vi "FeedbackDecode_GetPupilInfo.vi"(3 "FullDataPath":path=path "D:/FeedbackDecode/00000000-000000") -> ()   [LabVIEW 2020]
uses:
  <vilib>/addons/zeromq/socket_type.ctl
  <vilib>/addons/zeromq/socket_options.ctl
  <vilib>/DAQmx/write.llb/DAQmx Write (Analog DBL 1Chan 1Samp).vi
  FeedbackDecode_Globals.vi
  <vilib>/DAQmx/miscellaneous.llb/DAQmx Fill In Error Info.vi
  <vilib>/addons/zeromq/zeromq.lvlib
  <vilib>/addons/zeromq/zmq_context.lvclass
  <vilib>/addons/zeromq/zmq_socket.lvclass
panel:
  out "PupilDia":dbl
  out "PupilClust":T1
  out "error out":errorcluster
  out "RecStatus":string
  out "FileTime":string
  out "DataFolderName":string="00000000-000000"
  out "SubPort":string
  out "Acquire":dbl(graph)
  out "message":string[](array[string])
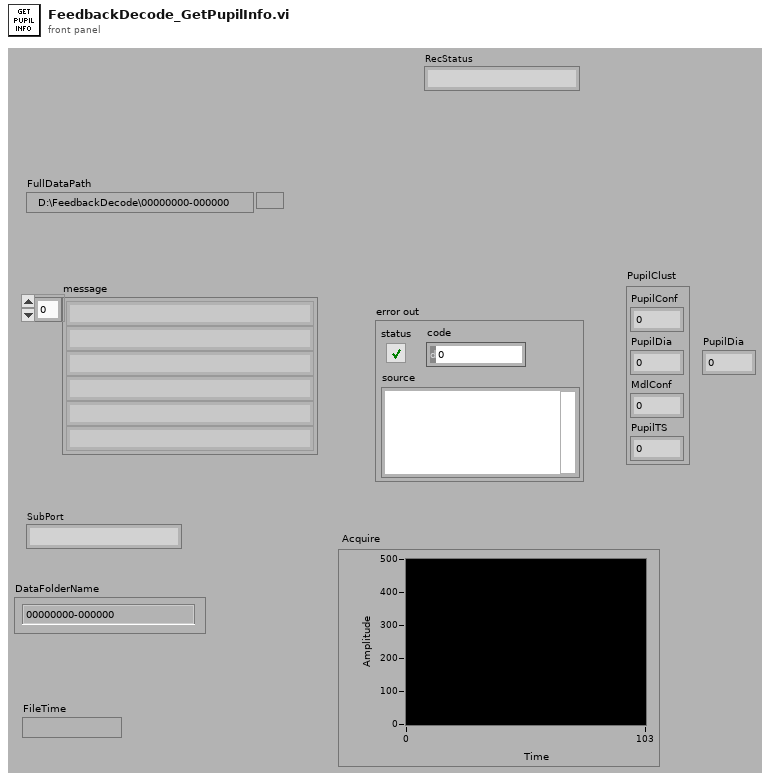
[diagram p1: front panel]
types:
  T1 = cluster{"PupilConf":dbl, "PupilDia":dbl, "MdlConf":dbl, "PupilTS":dbl}
  T2 = typedef "zeromq.lvlib/socket_options.ctl" = enum8{"NONE", "ZMQ_HWM", "<2>", "ZMQ_SWAP", "ZMQ_AFFINITY", "ZMQ_IDENTITY", "ZMQ_SUBSCRIBE", "ZMQ_UNSUBSCRIBE", "ZMQ_RATE", "ZMQ_RECOVERY_IVL", "ZMQ_MCAST_LOOP", "ZMQ_SNDBUF", "ZMQ_RCVBUF", "ZMQ_RCVMORE", "ZMQ_FD", "ZMQ_EVENTS", "ZMQ_TYPE", "ZMQ_LINGER", "ZMQ_RECONNECT_IVL", "ZMQ_BACKLOG", "ZMQ_RECOVERY_IVL_MSEC", "ZMQ_RECONNECT_IVL_MAX", "ZMQ_MAXMSGSIZE", "ZMQ_SNDHWM", "ZMQ_RCVHWM", "ZMQ_MULTICAST_HOPS", "<26>", "ZMQ_RCVTIMEO", "ZMQ_SNDTIMEO", "<29>", "<30>", "ZMQ_IPV4ONLY", "ZMQ_LAST_ENDPOINT", "ZMQ_ROUTER_MANDATORY", "ZMQ_TCP_KEEPALIVE", "ZMQ_TCP_KEEPALIVE_CNT", "ZMQ_TCP_KEEPALIVE_IDLE", "ZMQ_TCP_KEEPALIVE_INTVL", "ZMQ_TCP_ACCEPT_FILTER", "ZMQ_DELAY_ATTACH_ON_CONNECT", "ZMQ_XPUB_VERBOSE"}
  T3 = typedef "zeromq.lvlib/socket_type.ctl" = enum8{"ZMQ_PAIR", "ZMQ_PUB", "ZMQ_SUB", "ZMQ_REQ", "ZMQ_REP", "ZMQ_DEALER", "ZMQ_ROUTER", "ZMQ_PULL", "ZMQ_PUSH", "ZMQ_XPUB", "ZMQ_XSUB"}
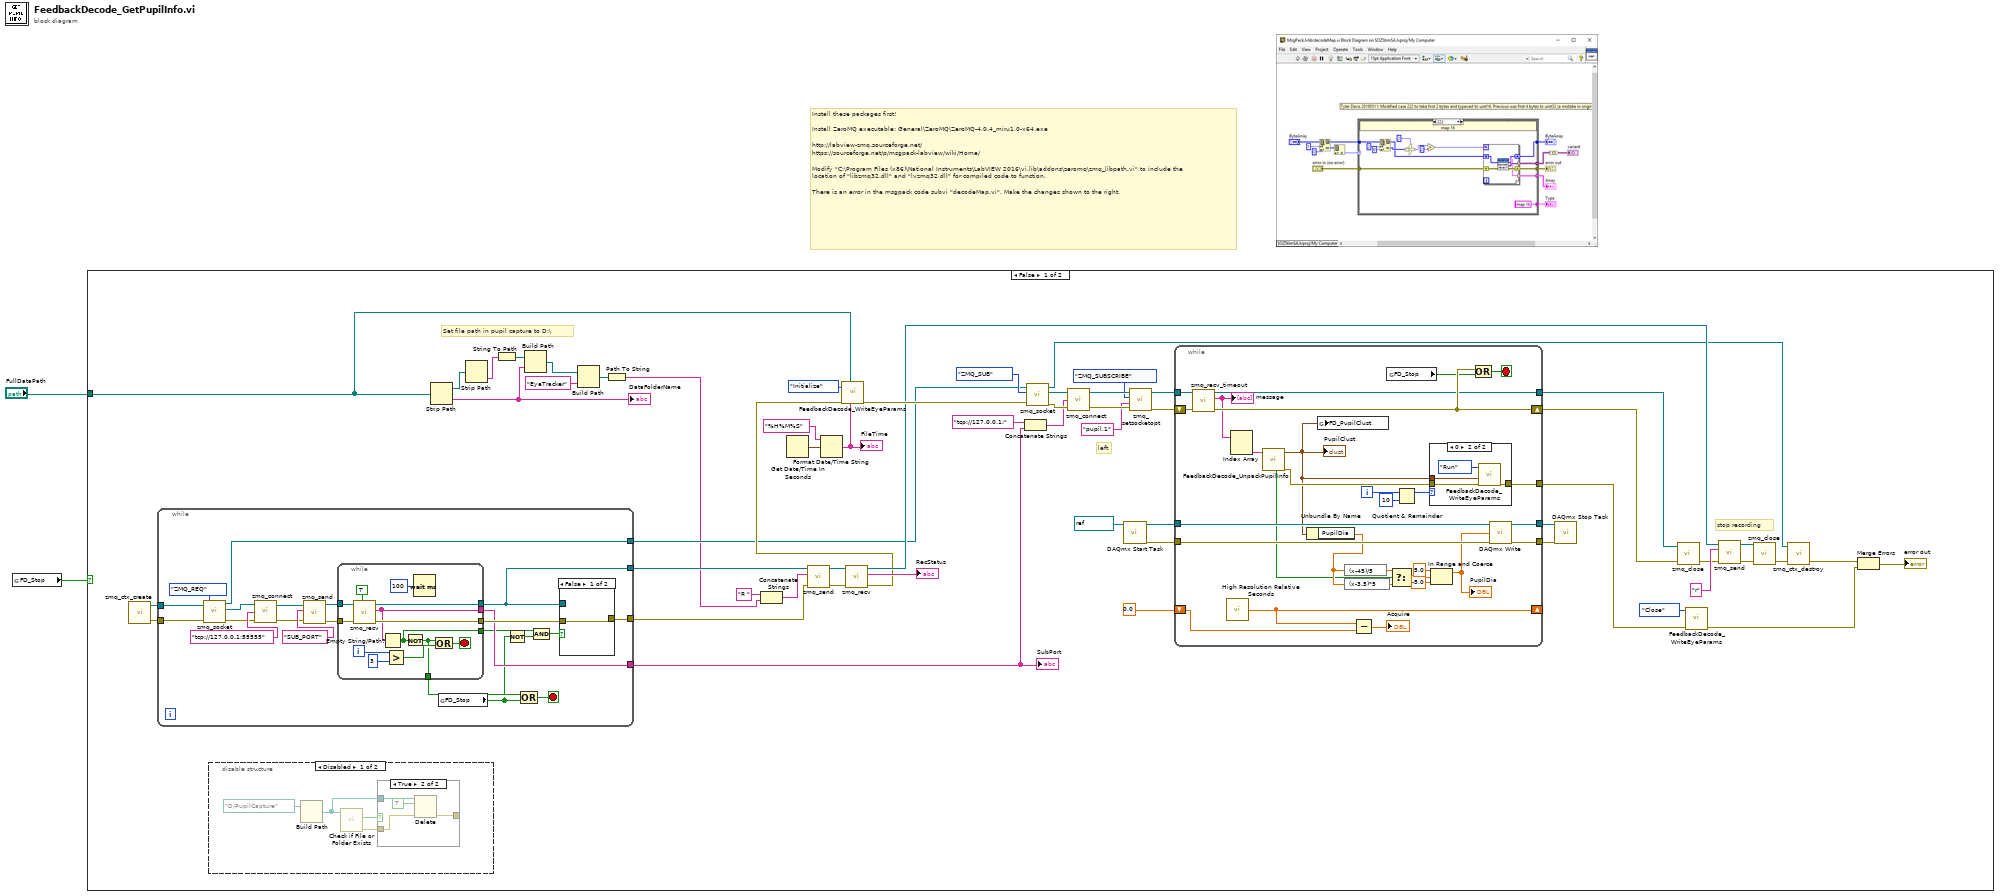
[diagram p0: block diagram]
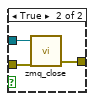
[diagram p2: hidden frame]
diagram:
  # "Install these packages first!\n\nInstall ZeroMQ executable: General\\ZeroMQ\\ZeroMQ-4.0.4_miru1.0-x64.exe\n\nhttp://labview-zmq.sourceforge.net/\nhttps://sourceforge.net/p/msgpack-labview/wiki/Home/\n\nModify \"C:\\Program Files (x86)\\National Instruments\\LabVIEW 2016\\vi.lib\\addons\\zeromq\\zmq_libpath.vi\" to include the location of \"libzmq32.dll\" and \"lvzmq32.dll\" for compiled code to function.\n\nThere is an error in the msgpack code subvi \"decodeMap.vi\". Make the changes shown to the right."
  n1 = global read "FeedbackDecode_Globals.vi" "FD_Stop"() -> (w1:bool)
  n2 = case shown="False" w1 {
    tunnel: "FullDataPath" -> [w5 _]
    frame False {
      # "Set file path in pupil capture to D:\\"
      # "left"
      # "stop recording"
      n3 = call <vilib>:"zmq_ctx_create.vi"() -> ("error out"=w21:errorcluster, "context out"=w22:refnum<class "zmq_context.lvclass">)  [unwired: 4 in]
      n4 = while {
        tunnel: [w72] -> w24
        tunnel: [w71] -> w23
        tunnel: [w67] -> w25
        tunnel: [w66] -> w20
        tunnel: w21 -> [w65]
        tunnel: w22 -> [w64]
        stop <- w78 stop-if-true
        n5 = call <vilib>:"zmq_socket.vi"("error in"=w65, "socket type"=socket_type."ZMQ_REQ", "context in"=w64) -> ("error out"=w69:errorcluster, "socket out"=w68:refnum<class "zmq_socket.lvclass">, "context out"=w66:refnum<class "zmq_context.lvclass">)  [unwired: 2 in]
        n6 = call <vilib>:"zmq_connect.vi"("error in"=w69, "endpoint"="tcp://127.0.0.1:55555", "socket in"=w68) -> ("error out"=w74:errorcluster, "socket out"=w75:refnum<class "zmq_socket.lvclass">)  [unwired: 1 in]
        n7 = call <vilib>:"zmq_send.vi"("error in"=w74, "data"="SUB_PORT", "socket in"=w75) -> ("error out"=w80:errorcluster, "socket out"=w79:refnum<class "zmq_socket.lvclass">)  [unwired: 4 in]
        n8 = while {
          tunnel: [w89] -> w71
          tunnel: [w87] -> w77
          tunnel: w79 -> [w97]
          tunnel: [w96] -> w67
          tunnel: w80 -> [w98]
          tunnel: [w95] -> w73
          tunnel: [w86] -> w63
          i -> [w90]
          stop <- w91 stop-if-true
          n9 = call <vilib>:"zmq_recv.vi"("no block? (F)"=TRUE, "error in"=w98, "socket in"=w97) -> ("error out"=w95:errorcluster, "data"=w89:string, "socket out"=w96:refnum<class "zmq_socket.lvclass">)  [unwired: 2 in, 2 out]
          n10 = Empty String/Path?(string/path=w89) -> (empty?=w86:bool)
          n11 = Greater?(x=w90, y=3) -> (0:w88:bool)
          n12 = Not(x=w86) -> (.not. x?=w87:bool)
          n13 = Wait (ms)(milliseconds to wait=u32 100) -> ()  [unwired: 1 out]
          n14 = Compound Arithmetic op=OR(w87, w88) -> (w91:bool)
        }
        n15 = global read "FeedbackDecode_Globals.vi" "FD_Stop"() -> (w60:bool)
        n16 = Not(x=w60) -> (.not. x?=w62:bool)
        n17 = Compound Arithmetic op=OR(w77, w60) -> (w78:bool)
        n18 = Compound Arithmetic op=AND(w63, w62) -> (w61:bool)
        n19 = case shown="False" w61 {
          tunnel: w67 -> [_ w85]
          tunnel: w73 -> [w82 w84]
          tunnel: [w82 w83] -> w72
          frame False {
          }
          frame True {
            n20 = call <vilib>:"zmq_close.vi"("error in"=w84, "socket"=w85) -> ("error out"=w83:errorcluster)  [unwired: 3 in]
          }
        }
      }
      "SubPort" <- w23
      n21 = disable-structure shown="Disabled" {
        frame Disabled {
          n22 = Build Path(base path=path "D:/PupilCapture") -> (appended path=w100:path)  [unwired: 1 in]
          n23 = call <vilib>:"Check if File or Folder Exists.vi"("path"=w100) -> ("error out"=w99:errorcluster, "file or folder exists?"=w101:bool)  [unwired: 8 in, 1 out]
          n24 = case shown="True" w101 {
            tunnel: w100 -> [_ w107]
            tunnel: w99 -> [w103 w106]
            tunnel: [w103 w105] -> _
            frame False {
            }
            frame True {
              n25 = Delete(path (use dialog)=w107, entire hierarchy (F)=TRUE, error in=w106) -> (error out=w105:errorcluster)  [unwired: 2 in, 2 out]
            }
          }
        }
        frame Enabled {
        }
      }
      n26 = Strip Path(path=w5) -> (stripped path=w6:path, name=w4:string)
      "DataFolderName" <- w4
      n27 = Strip Path(path=w6) -> (name=w7:string)  [unwired: 1 out]
      n28 = String To Path(string=w7) -> (path=w8:path)
      n29 = Build Path(base path=w8, name or relative path=w4) -> (appended path=w9:path)
      n30 = Build Path(base path=w9, name or relative path="EyeTracker") -> (appended path=w11:path)
      n31 = Path To String(path=w11) -> (string=w3:string)
      n32 = Concatenate Strings("R " ("data"), w3) -> (w48:string)
      n33 = Get Date/Time In Seconds() -> (seconds since 1Jan1904=w56:timestamp)
      n34 = call <vilib>:"zmq_send.vi"("error in"=w24, "data"=w48, "socket in"=w25) -> ("error out"=w54:errorcluster, "socket out"=w53:refnum<class "zmq_socket.lvclass">)  [unwired: 4 in]
      n35 = Format Date/Time String(time format string (%c)="%H%M%S", seconds (now)=w56) -> (date/time string=w49:string)  [unwired: 1 in]
      "FileTime" <- w49
      n36 = call <vilib>:"zmq_recv.vi"("error in"=w54, "socket in"=w53) -> ("error out"=w51:errorcluster, "data"=→"RecStatus":string, "socket out"=w58:refnum<class "zmq_socket.lvclass">)  [unwired: 3 in, 2 out]
      n37 = call "FeedbackDecode_WriteEyeParams.vi"("FileTime"=w49, "DataPath"=w5, "ErrorIn"=w51, "Mode"=enum16{"Initialize", "Run", "Close"}."Initialize") -> ("ErrorOut"=w59:errorcluster)  [unwired: 6 in, 1 out]
      n38 = Concatenate Strings("tcp://127.0.0.1:" ("endpoint"), w23) -> (w38:string)
      n39 = call <vilib>:"zmq_socket.vi"("error in"=w59, "socket type"=socket_type."ZMQ_SUB", "context in"=w20) -> ("error out"=w46:errorcluster, "socket out"=w40:refnum<class "zmq_socket.lvclass">, "context out"=w32:refnum<class "zmq_context.lvclass">)  [unwired: 2 in]
      n40 = call <vilib>:"zmq_connect.vi"("error in"=w46, "endpoint"=w38, "socket in"=w40) -> ("error out"=w44:errorcluster, "socket out"=w45:refnum<class "zmq_socket.lvclass">)  [unwired: 1 in]
      n41 = call <vilib>:"DAQmx Start Task.vi"("task/channels in"=refnum<k21> "Pupil") -> ("task out"=w15:refnum<k21>, "error out"=w14:errorcluster)  [unwired: 13 in]
      n42 = call <vilib>:"zmq_setsocketopt.vi"("error in"=w44, "value"="pupil.1", "option"=socket_options."ZMQ_SUBSCRIBE", "socket in"=w45) -> ("error out"=w36:errorcluster, "socket out"=w43:refnum<class "zmq_socket.lvclass">)  [unwired: 2 in]
      n43 = while {
        tunnel: w43 -> [w136]
        shift-right: [w125] -> _
        shift-left: 0.0 -> [w134]
        shift-right: [w132] -> w19
        shift-left: w36 -> [w135]
        tunnel: [w130] -> w33
        tunnel: [w126] -> w17
        tunnel: w15 -> [w121]
        tunnel: w14 -> [w120]
        tunnel: [w119] -> w13
        tunnel: [w118] -> w12
        i -> [w123]
        stop <- w131 stop-if-true
        n44 = call <vilib>:"zmq_recv_timeout.vi"("error in"=w135, "socket in"=w136) -> ("error out"=w132:errorcluster, "parts"=w127:string[], "socket out"=w130:refnum<class "zmq_socket.lvclass">)  [unwired: 2 in, 1 out]
        "message" <- w127
        n45 = call <vilib>:"High Resolution Relative Seconds.vi"() -> ("relative seconds"=w125:dbl)
        n46 = Index Array(array=w127) -> (element #2=w128:string)  [unwired: 2 in, 1 out]
        n47 = call "FeedbackDecode_UnpackPupilInfo.vi"("MSGPackStr"=w128) -> ("ErrorOut"=w129:errorcluster, "PupilClust"=w109:T1, "Pupil2d"=w111:bool)  [unwired: 8 in]
        "PupilClust" <- w109
        n48 = Unbundle By Name(w109) -> ("PupilDia"=w112:dbl)
        n49 = global write "FeedbackDecode_Globals.vi" "FD_PupilClust"(w109) -> ()
        n50 = expression code="(x-45)/5"(w112) -> (w117:dbl)
        n51 = expression code="(x-3.5)*5"(w112) -> (w116:dbl)
        n52 = Subtract(x=w125, y=w134) -> (x-y=→"Acquire":dbl)
        n53 = global read "FeedbackDecode_Globals.vi" "FD_Stop"() -> (w108:bool)
        n54 = Select(t=w117, s=w111, f=w116) -> (s? t:f=w115:dbl)
        n55 = Quotient & Remainder(x=w123, y=10) -> (x-y*floor(x/y)=w124:i32)  [unwired: 1 out]
        n56 = case shown="0" w124 {
          tunnel: w109 -> [_ w141]
          tunnel: w129 -> [w137 w140]
          tunnel: [w137 w139] -> w126
          frame 1, Default {
          }
          frame 0 {
            n57 = call "FeedbackDecode_WriteEyeParams.vi"("ErrorIn"=w140, "PupilClust"=w141, "Mode"=enum16{"Initialize", "Run", "Close"}."Run") -> ("ErrorOut"=w139:errorcluster)  [unwired: 7 in, 1 out]
          }
        }
        n58 = In Range and Coerce(upper limit=5.0, x=w115, lower limit=-5.0) -> (coerced(x)=w110:dbl)  [unwired: 1 out]
        "PupilDia" <- w110
        n59 = Compound Arithmetic op=OR(w132, w108) -> (w131:bool)
        n60 = call-poly <vilib>:"DAQmx Write.vi"("task/channels in"=w121, "data"=w110, "error in"=w120) -> ("task out"=w119:refnum<k21>, "error out"=w118:errorcluster)  [unwired: 10 in, 1 out]
      }
      n61 = call <vilib>:"DAQmx Stop Task.vi"("task/channels in"=w13, "error in"=w12) -> ()  [unwired: 12 in, 2 out]
      n62 = call <vilib>:"zmq_close.vi"("error in"=w19, "socket"=w33) -> ("error out"=w31:errorcluster)  [unwired: 3 in]
      n63 = call "FeedbackDecode_WriteEyeParams.vi"("ErrorIn"=w17, "Mode"=enum16{"Initialize", "Run", "Close"}."Close") -> ("ErrorOut"=w18:errorcluster)  [unwired: 8 in, 1 out]
      n64 = call <vilib>:"zmq_send.vi"("error in"=w31, "data"="r", "socket in"=w58) -> ("error out"=w26:errorcluster, "socket out"=w27:refnum<class "zmq_socket.lvclass">)  [unwired: 4 in]
      n65 = call <vilib>:"zmq_close.vi"("error in"=w26, "socket"=w27) -> ("error out"=w30:errorcluster)  [unwired: 3 in]
      n66 = call <vilib>:"zmq_ctx_destroy.vi"("error in"=w30, "context in"=w32) -> ("error out"=w29:errorcluster)  [unwired: 3 in]
      n67 = Merge Errors(w29, w18) -> (→"error out":errorcluster)
    }
    frame True {
    }
  }
